vi "Calculate Joystick Angle.vi"(1 "Joystick Y":dbl, 2 "Joystick X":dbl) -> (0 "Angle (radians)":dbl)   [LabVIEW 2016]
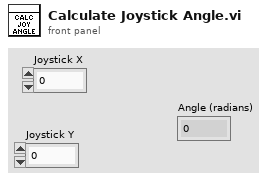
[diagram p1: front panel]
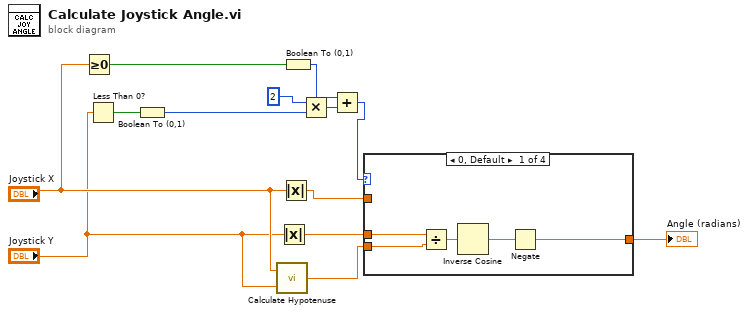
[diagram p0: block diagram]
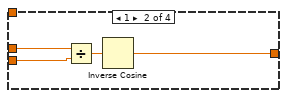
[diagram p2: hidden frame]
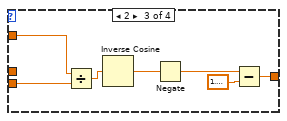
[diagram p3: hidden frame]
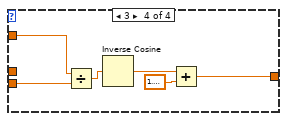
[diagram p4: hidden frame]
diagram:
  n1 = Greater Or Equal To 0?(x="Joystick X") -> (x >= 0?=w11:bool)
  n2 = Less Than 0?(x="Joystick Y") -> (x < 0?=w7:bool)
  n3 = Boolean To (0,1)(Boolean=w7) -> (0, 1=w6:i16)
  n4 = call "Calculate Hypotenuse.vi"("Y"="Joystick Y", "X"="Joystick X") -> ("Hypotenuse"=w4:dbl)
  n5 = Absolute Value(x="Joystick Y") -> (abs(x)=w5:dbl)
  n6 = Absolute Value(x="Joystick X") -> (abs(x)=w12:dbl)
  n7 = Boolean To (0,1)(Boolean=w11) -> (0, 1=w10:i16)
  n8 = Multiply(x=i16 2, y=w6) -> (x*y=w9:i16)
  n9 = Add(x=w10, y=w9) -> (x+y=w8:i16)
  n10 = case shown="0, Default" w8 {
    tunnel: w12 -> [_ _ w27 w34]
    tunnel: [w14 w19 w23 w30] -> w13
    tunnel: w5 -> [w17 w20 _ _]
    tunnel: w4 -> [w16 w21 w26 w33]
    frame 0, Default {
      n11 = Divide(x=w17, y=w16) -> (x/y=w18:dbl)
      n12 = Inverse Cosine(1:w18) -> (0:w15:dbl)
      n13 = Negate(x=w15) -> (-x=w14:dbl)
    }
    frame 1 {
      n14 = Divide(x=w20, y=w21) -> (x/y=w22:dbl)
      n15 = Inverse Cosine(1:w22) -> (0:w19:dbl)
    }
    frame 2 {
      n16 = Divide(x=w27, y=w26) -> (x/y=w29:dbl)
      n17 = Inverse Cosine(1:w29) -> (0:w28:dbl)
      n18 = Negate(x=w28) -> (-x=w25:dbl)
      n19 = Subtract(x=w25, y=1.5707963267948966) -> (x-y=w23:dbl)
    }
    frame 3 {
      n20 = Divide(x=w34, y=w33) -> (x/y=w35:dbl)
      n21 = Inverse Cosine(1:w35) -> (0:w32:dbl)
      n22 = Add(x=w32, y=1.5707963267948966) -> (x+y=w30:dbl)
    }
  }
  "Angle (radians)" <- w13
